vi "Yokogawa - write file.vi"(8 "error in (no error)":errorcluster, 10 "Electrical Data 2":T1, 11 "Metadata":string[][](array[string])) -> (0 "error out":errorcluster, 3 "file path out":path)   [LabVIEW 2013]
uses:
  electrical2.ctl
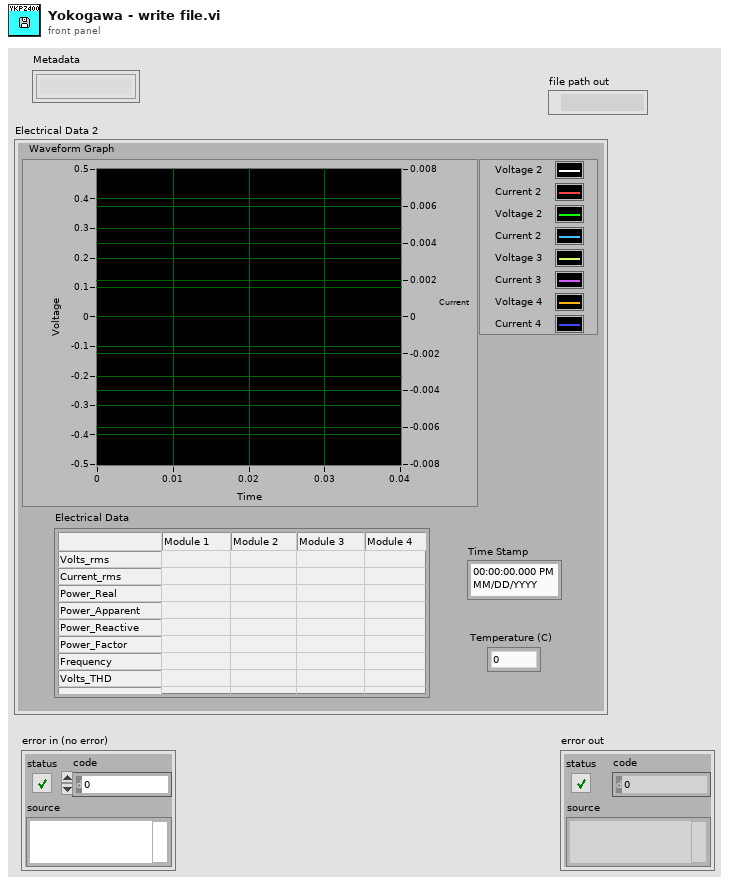
[diagram p1: front panel]
types:
  T1 = typedef "electrical2.ctl" = cluster{"Time Stamp":timestamp, "Temperature (C)":dbl, "Electrical Data":string[][], "Waveform Graph":waveform(dbl)[]}
  T2 = enum16{"open", "open or create", "create or replace", "create", "open (read-only)"}
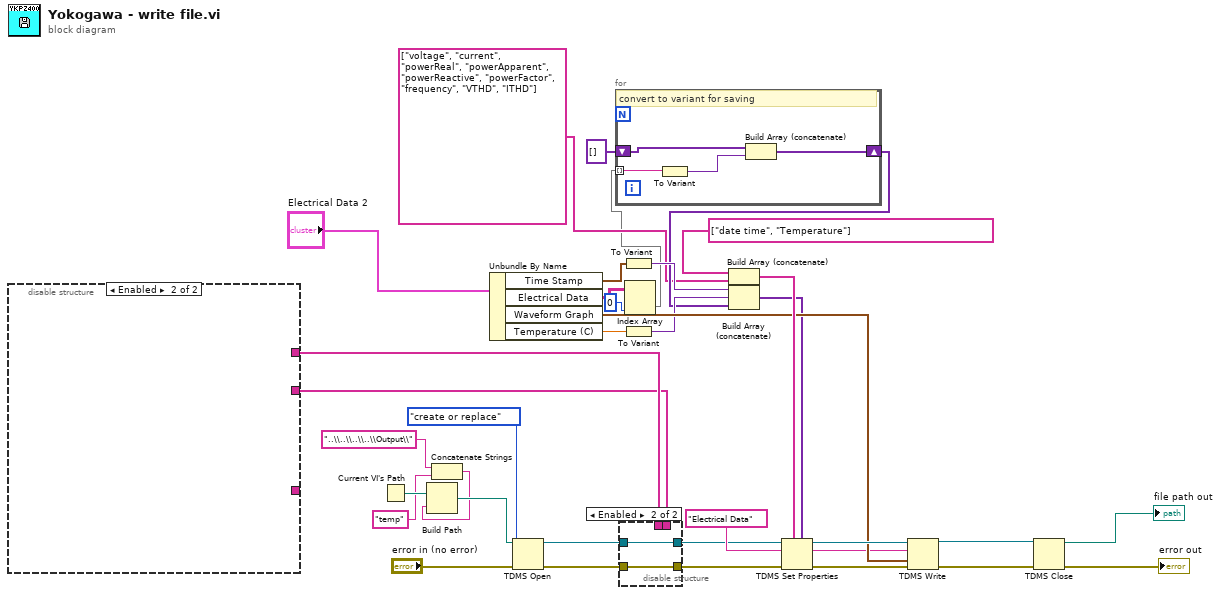
[diagram p0: block diagram]
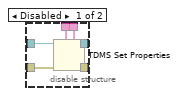
[diagram p2: hidden frame]
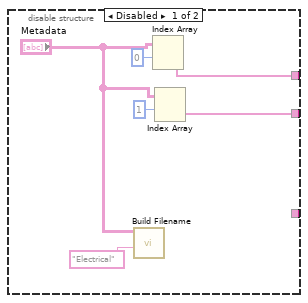
[diagram p3: hidden frame]
diagram:
  n1 = disable-structure shown="Enabled" {
    disable-tunnel: [w40 _] -> w18
    disable-tunnel: [w39 _] -> w17
    disable-tunnel: _ -> [w37 _]
    frame Disabled {
      n2 = call "Build Filename.vi"("Measurment Type"="Electrical", "Metadata In"="Metadata") -> ()  [unwired: 9 in, 1 out]
      n3 = Index Array(array="Metadata", index (row)=0) -> (element=w40:string[])  [unwired: 1 in]
      n4 = Index Array(array="Metadata", index (row)=1) -> (element=w39:string[])  [unwired: 1 in]
    }
    frame Enabled {
    }
  }
  n5 = Current VI's Path() -> (path=w27:path)
  n6 = Concatenate Strings("..\\..\\..\\..\\Output\\" ("string"), "temp" ("name or relative path")) -> (w4:string)
  n7 = Build Path(base path=w27, name or relative path=w4) -> (appended path=w26:path)
  n8 = Unbundle By Name("Electrical Data 2") -> ("Time Stamp"=w9:timestamp, "Electrical Data"=w2:string[][], "Waveform Graph"=w30:waveform(dbl)[], "Temperature (C)"=w16:dbl)
  n9 = TDMS Open(8:"error in (no error)", 10:T2."create or replace" ("operation (0:open)"), 11:w26) -> (0:w21:errorcluster, 3:w22:refnum<k34>)  [unwired: 4 in]
  n10 = disable-structure shown="Enabled" {
    disable-tunnel: w22 -> [w49 w51]
    disable-tunnel: w21 -> [w48 w50]
    disable-tunnel: [w47 w51] -> w20
    disable-tunnel: [w46 w50] -> w19
    disable-tunnel: w18 -> [w45 _]
    disable-tunnel: w17 -> [w44 _]
    frame Disabled {
      n11 = TDMS Set Properties(5:w44, 7:w45, 8:w48, 11:w49) -> (0:w46:errorcluster, 3:w47:refnum<k34>)  [unwired: 2 in, 2 out]
    }
    frame Enabled {
    }
  }
  n12 = To Variant(anything=w9) -> (Variant=w14:variant)
  n13 = To Variant(anything=w16) -> (Variant=w13:variant)
  n14 = Index Array(array=w2, index (col)=0 ("index (row)")) -> (element=w3:string[])  [unwired: 1 in]
  n15 = for {
    tunnel: w3 -> [w55] mode=indexing
    shift-right: [w54] -> w12
    shift-left: variant[] [] -> [w52]
    # "convert to variant for saving"
    n16 = To Variant(anything=w55) -> (Variant=w53:variant)
    n17 = Build Array (concatenate)(w52, w53) -> (w54:variant[])
  }
  n18 = Build Array (concatenate)(string[] ["date time", "Temperature"] ("element"), string[] ["voltage", "current", "powerReal", "powerApparent", "powerReactive", "powerFactor", "frequency", "VTHD", "ITHD"]) -> (w31:string[])
  n19 = Build Array (concatenate)(w14, w13, w12) -> (w15:variant[])
  n20 = TDMS Set Properties(5:w15, 7:w31, 8:w19, 10:"Electrical Data" ("group name"), 11:w20) -> (0:w35:errorcluster, 2:w23:string, 3:w36:refnum<k34>)  [unwired: 1 in, 1 out]
  n21 = TDMS Write(0:w36, 5:w23, 9:w30, 11:w35) -> (4:w34:refnum<k34>, 15:w33:errorcluster)  [unwired: 2 in, 2 out]
  n22 = TDMS Close(8:w33, 11:w34) -> (0:→"error out":errorcluster, 3:→"file path out":path)
